vi "loggin'.vi"() -> ()   [LabVIEW 2018]
uses:
  <vilib>/Platform/TimedLoop/XDataNode/wakeup.ctl
  <vilib>/Platform/TimedLoop/XDataNode/XDNodeRunTimeDep.lvlib
  <vilib>/Platform/TimedLoop/XDataNode/nitl_modes.ctl
  <vilib>/Platform/TimedLoop/XDataNode/timing_clust.ctl
  <vilib>/platform/TimedLoop/XDataNode/XDataNode.xnode
  <userlib>/836-Library/System/QCP_V2/QCPSupportCode/QCPData.ctl
panel:
  out "QCP Finished Late? [i-1]":bool
  out "QCP Iteration Duration":i64=10
  in  "QCPPeriod":i64=100
  in  "DriveWriteQCPFile":bool
  in  "AutoWriteQCPFile":bool
  in  "HatchPanelWriteQCPFile":bool
  in  "ClimbWriteQCPFile":bool
  in  "CargoWriteQCPFile":bool
  in  "LiftTuningMode?":bool=TRUE
  in  "DriveTuningMode?":bool=TRUE
  in  "AutoTuningMode?":bool
  in  "IntakeTuningMode?":bool=TRUE
  in  "SensorTuningMode?":bool
  in  "Read Lift QCP":bool
  in  "Read Drive QCP":bool
  in  "Read Auto QCP":bool
  in  "Read Sensor QCP":bool
  in  "Read Intake QCP":bool
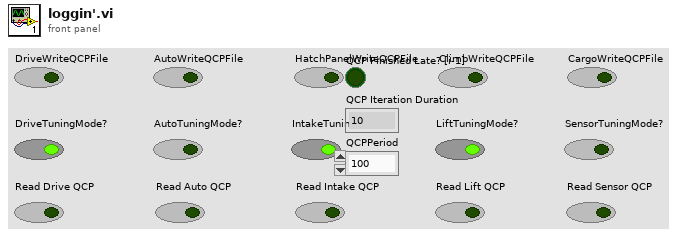
[diagram p1: front panel]
types:
  T1 = typedef "XDNodeRunTimeDep.lvlib/timing_clust.ctl" = cluster{"Expected End [f-1]":u64, "Actual End [f-1]":u64, "Finished Late? [f-1]":bool, "Expected End [i-1]":u64, "Actual End [i-1]":u64, "Finished Late? [i-1]":bool, "Expected Start [i]":u64, "Actual Start [i]":u64, "Expected Start [f]":u64, "Actual Start [f]":u64, "Source Name":string, "Structure Name":string, "Period":i64, "Deadline":i64, "Offset":i64, "Start":i64, "Priority":i32, "Timeout":i32, "Mode":T2, "Wakeup Reason":T3, "Error":errorcluster, "Source Type":string, "Secondary Source Type":string, "Global End Time":u64, "Global Start Time":u64, "Frame Duration":u64, "Iteration Duration":u64, "Assigned CPU":i32, "I/O Scan Engine Mode":u32}
  T2 = typedef "XDNodeRunTimeDep.lvlib/nitl_modes.ctl" = enum32{"No Change", "Process missed periods, maintain original phase", "Discard missed periods, maintain original phase", "Process missed periods, ignore original phase", "Discard missed periods, ignore original phase"}
  T3 = typedef "XDNodeRunTimeDep.lvlib/wakeup.ctl" = enum32{"Normal", "Aborted", "Asynchronous wakeup", "Timing source error", "Timed loop error", "Timeout"}
  T4 = typedef "Semaphore RefNum" = refnum<k1>
  T5 = cluster{"Data Value Refnum":refnum<data-value>, "semaphore":T4}
  T6 = typedef "QCP_RefNum.ctl" = cluster{"Data Value Refnum":refnum<data-value>, "semaphore":T4}
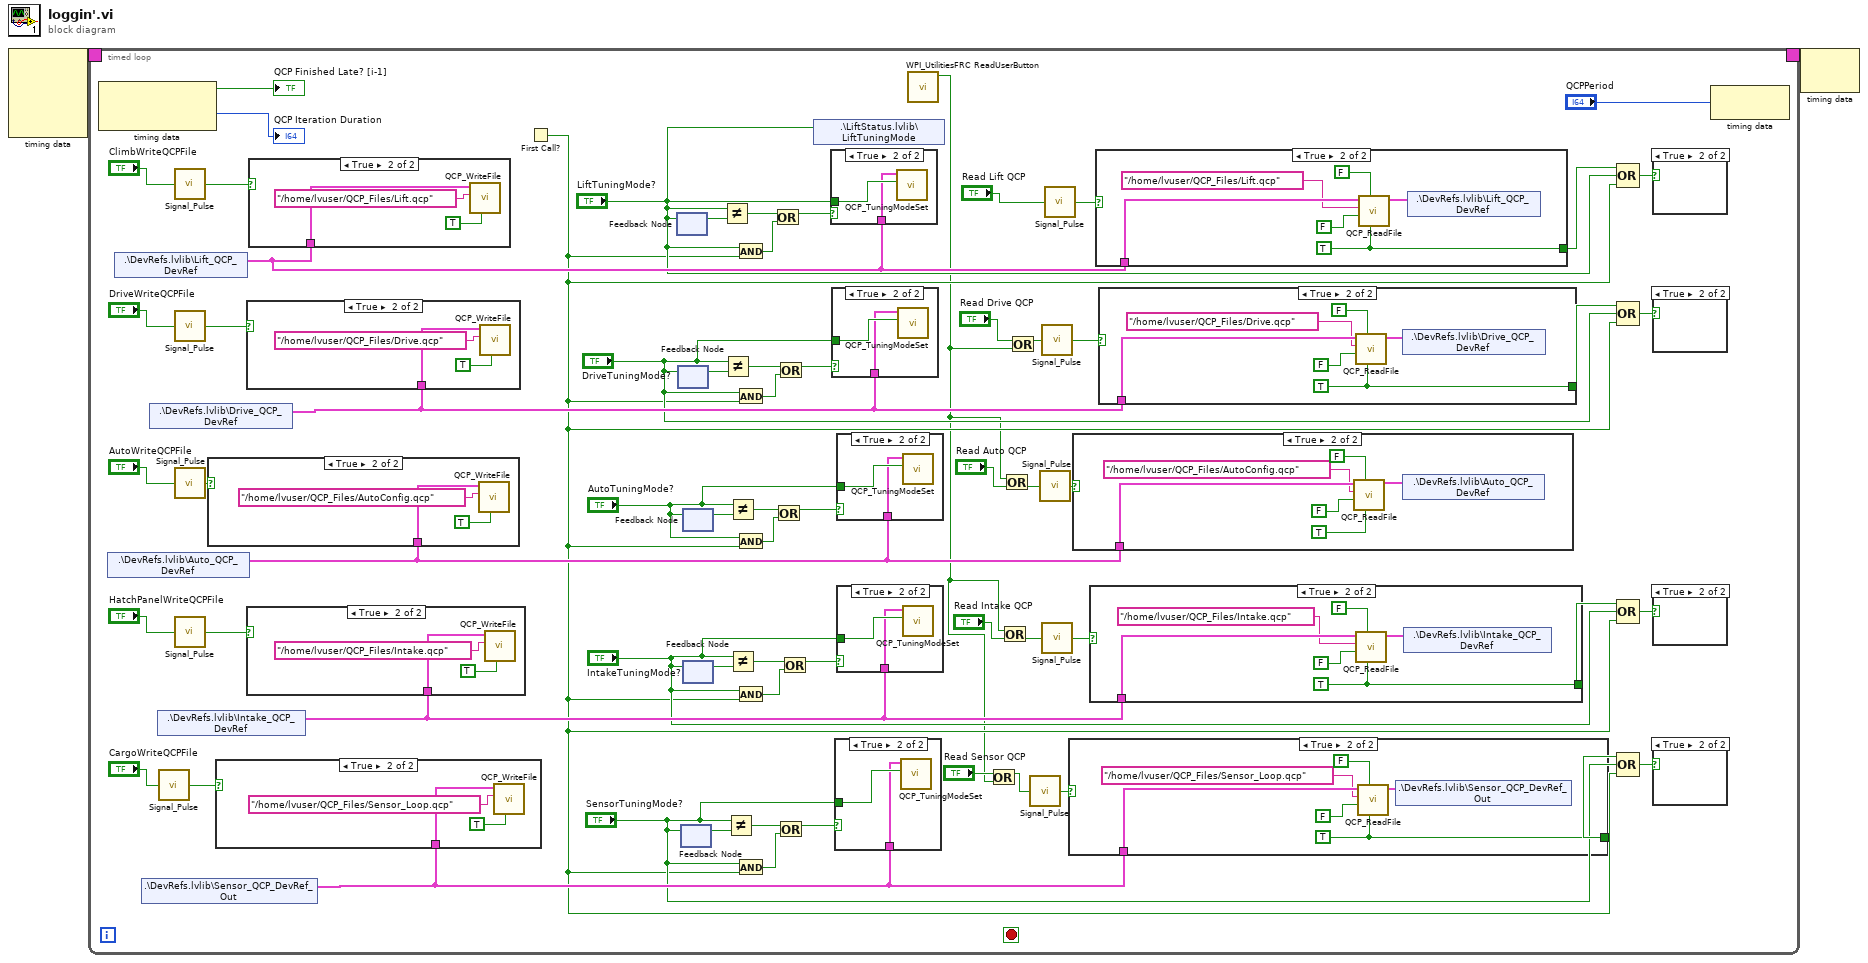
[diagram p0: block diagram]
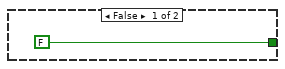
[diagram p6: hidden frame]
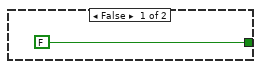
[diagram p7: hidden frame]
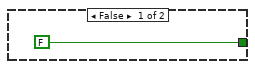
[diagram p9: hidden frame]
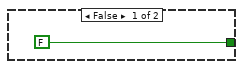
[diagram p10: hidden frame]
diagram:
  n1 = node-c288() -> (w2:T1)  [unwired: 4 in]
  n2 = timed-loop {
    timing: w2 -> [_]
    timing-out: [_] -> w1
    stop <- _ stop-if-true
    n3 = node-c288() -> (→"QCP Finished Late? [i-1]":bool, →"QCP Iteration Duration":i64)  [unwired: 1 in]
    n4 = shared-variable ".\\DevRefs.lvlib\\Auto_QCP_DevRef"() -> (w28:T5)  [unwired: 1 in, 1 out]
    n5 = shared-variable ".\\DevRefs.lvlib\\Lift_QCP_DevRef"() -> (w30:T5)  [unwired: 1 in, 1 out]
    n6 = shared-variable ".\\DevRefs.lvlib\\Sensor_QCP_DevRef_Out"() -> (w27:T5)  [unwired: 1 in, 1 out]
    n7 = shared-variable ".\\DevRefs.lvlib\\Drive_QCP_DevRef"() -> (w29:T5)  [unwired: 1 in, 1 out]
    n8 = shared-variable ".\\DevRefs.lvlib\\Intake_QCP_DevRef"() -> (w31:T5)  [unwired: 1 in, 1 out]
    n9 = call <userlib>:"Signal_Pulse.vi"("Input"="CargoWriteQCPFile") -> ("Output"=w58:bool)
    n10 = call <userlib>:"Signal_Pulse.vi"("Input"="ClimbWriteQCPFile") -> ("Output"=w60:bool)
    n11 = call <userlib>:"Signal_Pulse.vi"("Input"="DriveWriteQCPFile") -> ("Output"=w66:bool)
    n12 = call <userlib>:"Signal_Pulse.vi"("Input"="AutoWriteQCPFile") -> ("Output"=w64:bool)
    n13 = call <userlib>:"Signal_Pulse.vi"("Input"="HatchPanelWriteQCPFile") -> ("Output"=w62:bool)
    n14 = case shown="True" w64 {
      tunnel: w28 -> [_ w124]
      frame False {
      }
      frame True {
        n15 = call <userlib>:"QCP_WriteFile.vi"("Overrite?"=TRUE, "Path"="/home/lvuser/QCP_Files/AutoConfig.qcp", "QCP_DevRef_In"=w124) -> ()  [unwired: 7 in, 2 out]
      }
    }
    n16 = case shown="True" w58 {
      tunnel: w27 -> [_ w115]
      frame False {
      }
      frame True {
        n17 = call <userlib>:"QCP_WriteFile.vi"("Overrite?"=TRUE, "Path"="/home/lvuser/QCP_Files/Sensor_Loop.qcp", "QCP_DevRef_In"=w115) -> ()  [unwired: 7 in, 2 out]
      }
    }
    n18 = case shown="True" w66 {
      tunnel: w29 -> [_ w127]
      frame False {
      }
      frame True {
        n19 = call <userlib>:"QCP_WriteFile.vi"("Overrite?"=TRUE, "Path"="/home/lvuser/QCP_Files/Drive.qcp", "QCP_DevRef_In"=w127) -> ()  [unwired: 7 in, 2 out]
      }
    }
    n20 = case shown="True" w62 {
      tunnel: w31 -> [_ w121]
      frame False {
      }
      frame True {
        n21 = call <userlib>:"QCP_WriteFile.vi"("Overrite?"=TRUE, "Path"="/home/lvuser/QCP_Files/Intake.qcp", "QCP_DevRef_In"=w121) -> ()  [unwired: 7 in, 2 out]
      }
    }
    n22 = case shown="True" w60 {
      tunnel: w30 -> [_ w118]
      frame False {
      }
      frame True {
        n23 = call <userlib>:"QCP_WriteFile.vi"("Overrite?"=TRUE, "Path"="/home/lvuser/QCP_Files/Lift.qcp", "QCP_DevRef_In"=w118) -> ()  [unwired: 7 in, 2 out]
      }
    }
    n24 = First Call?() -> (First Call?: T/F=w10:bool)
    n25 = feedback #1() -> (w56:bool)  [unwired: 1 in]
    n26 = feedback-in #1("LiftTuningMode?") -> ()
    n27 = feedback #2() -> (w55:bool)  [unwired: 1 in]
    n28 = feedback-in #2("DriveTuningMode?") -> ()
    n29 = feedback #3() -> (w49:bool)  [unwired: 1 in]
    n30 = feedback-in #3("SensorTuningMode?") -> ()
    n31 = feedback #4() -> (w53:bool)  [unwired: 1 in]
    n32 = feedback-in #4("AutoTuningMode?") -> ()
    n33 = feedback #5() -> (w51:bool)  [unwired: 1 in]
    n34 = feedback-in #5("IntakeTuningMode?") -> ()
    n35 = Not Equal?(x="LiftTuningMode?", y=w56) -> (x != y?=w21:bool)
    n36 = Not Equal?(x="DriveTuningMode?", y=w55) -> (x != y?=w54:bool)
    n37 = Not Equal?(x="SensorTuningMode?", y=w49) -> (x != y?=w48:bool)
    n38 = Not Equal?(x="AutoTuningMode?", y=w53) -> (x != y?=w52:bool)
    n39 = Not Equal?(x="IntakeTuningMode?", y=w51) -> (x != y?=w50:bool)
    n40 = And(x="LiftTuningMode?", y=w10) -> (x .and. y?=w20:bool)
    n41 = And(x="DriveTuningMode?", y=w10) -> (x .and. y?=w18:bool)
    n42 = And(x="AutoTuningMode?", y=w10) -> (x .and. y?=w11:bool)
    n43 = And(x="IntakeTuningMode?", y=w10) -> (x .and. y?=w15:bool)
    n44 = And(x="SensorTuningMode?", y=w10) -> (x .and. y?=w13:bool)
    n45 = Or(x=w21, y=w20) -> (x .or. y?=w22:bool)
    n46 = Or(x=w52, y=w11) -> (x .or. y?=w24:bool)
    n47 = Or(x=w54, y=w18) -> (x .or. y?=w23:bool)
    n48 = Or(x=w48, y=w13) -> (x .or. y?=w26:bool)
    n49 = Or(x=w50, y=w15) -> (x .or. y?=w25:bool)
    n50 = shared-variable ".\\LiftStatus.lvlib\\LiftTuningMode"("LiftTuningMode?") -> ()  [unwired: 1 in, 1 out]
    n51 = case shown="True" w22 {
      tunnel: "LiftTuningMode?" -> [_ w113]
      tunnel: w30 -> [_ w112]
      frame False {
      }
      frame True {
        n52 = call <userlib>:"QCP_TuningModeSet.vi"("On?"=w113, "QCP_DevRef_In"=w112) -> ()  [unwired: 8 in, 2 out]
      }
    }
    n53 = case shown="True" w23 {
      tunnel: "DriveTuningMode?" -> [_ w111]
      tunnel: w29 -> [_ w110]
      frame False {
      }
      frame True {
        n54 = call <userlib>:"QCP_TuningModeSet.vi"("On?"=w111, "QCP_DevRef_In"=w110) -> ()  [unwired: 8 in, 2 out]
      }
    }
    n55 = case shown="True" w26 {
      tunnel: "SensorTuningMode?" -> [_ w105]
      tunnel: w27 -> [_ w104]
      frame False {
      }
      frame True {
        n56 = call <userlib>:"QCP_TuningModeSet.vi"("On?"=w105, "QCP_DevRef_In"=w104) -> ()  [unwired: 8 in, 2 out]
      }
    }
    n57 = case shown="True" w24 {
      tunnel: "AutoTuningMode?" -> [_ w109]
      tunnel: w28 -> [_ w108]
      frame False {
      }
      frame True {
        n58 = call <userlib>:"QCP_TuningModeSet.vi"("On?"=w109, "QCP_DevRef_In"=w108) -> ()  [unwired: 8 in, 2 out]
      }
    }
    n59 = case shown="True" w25 {
      tunnel: "IntakeTuningMode?" -> [_ w107]
      tunnel: w31 -> [_ w106]
      frame False {
      }
      frame True {
        n60 = call <userlib>:"QCP_TuningModeSet.vi"("On?"=w107, "QCP_DevRef_In"=w106) -> ()  [unwired: 8 in, 2 out]
      }
    }
    n61 = call <vilib>:"WPI_UtilitiesFRC ReadUserButton.vi"() -> ("User Button"=w4:bool)  [unwired: 10 in, 1 out]
    n62 = Or(x="Read Sensor QCP", y=w4) -> (x .or. y?=w5:bool)
    n63 = Or(x=w4, y="Read Intake QCP") -> (x .or. y?=w6:bool)
    n64 = Or(x=w4, y="Read Auto QCP") -> (x .or. y?=w7:bool)
    n65 = Or(x="Read Drive QCP", y=w4) -> (x .or. y?=w9:bool)
    n66 = call <userlib>:"Signal_Pulse.vi"("Input"=w5) -> ("Output"=w43:bool)
    n67 = call <userlib>:"Signal_Pulse.vi"("Input"=w7) -> ("Output"=w45:bool)
    n68 = call <userlib>:"Signal_Pulse.vi"("Input"=w9) -> ("Output"=w46:bool)
    n69 = call <userlib>:"Signal_Pulse.vi"("Input"=w6) -> ("Output"=w44:bool)
    n70 = call <userlib>:"Signal_Pulse.vi"("Input"="Read Lift QCP") -> ("Output"=w47:bool)
    n71 = case shown="True" w43 {
      tunnel: w27 -> [_ w76]
      tunnel: [FALSE ("Overrite Existing Data?") w72] -> w36
      frame False {
      }
      frame True {
        w72 = TRUE ("Overrite Existing Data?")
        n72 = call <userlib>:"QCP_ReadFile.vi"("Overrite Existing Data?"=w72, "Same Name Fail?"=FALSE, "Path Relative?"=FALSE, "Path"="/home/lvuser/QCP_Files/Sensor_Loop.qcp", "QCP_DevRef_In"=w76) -> ("QCP_DevRef_Out"=w71:T6)  [unwired: 5 in, 1 out]
        n73 = shared-variable ".\\DevRefs.lvlib\\Sensor_QCP_DevRef_Out"(w71) -> ()  [unwired: 1 in, 1 out]
      }
    }
    n74 = case shown="True" w45 {
      tunnel: w28 -> [_ w89]
      frame False {
      }
      frame True {
        n75 = call <userlib>:"QCP_ReadFile.vi"("Overrite Existing Data?"=TRUE, "Same Name Fail?"=FALSE, "Path Relative?"=FALSE, "Path"="/home/lvuser/QCP_Files/AutoConfig.qcp", "QCP_DevRef_In"=w89) -> ("QCP_DevRef_Out"=w84:T6)  [unwired: 5 in, 1 out]
        n76 = shared-variable ".\\DevRefs.lvlib\\Auto_QCP_DevRef"(w84) -> ()  [unwired: 1 in, 1 out]
      }
    }
    n77 = case shown="True" w44 {
      tunnel: w31 -> [_ w83]
      tunnel: [FALSE ("Overrite Existing Data?") w79] -> w38
      frame False {
      }
      frame True {
        w79 = TRUE ("Overrite Existing Data?")
        n78 = call <userlib>:"QCP_ReadFile.vi"("Overrite Existing Data?"=w79, "Same Name Fail?"=FALSE, "Path Relative?"=FALSE, "Path"="/home/lvuser/QCP_Files/Intake.qcp", "QCP_DevRef_In"=w83) -> ("QCP_DevRef_Out"=w78:T6)  [unwired: 5 in, 1 out]
        n79 = shared-variable ".\\DevRefs.lvlib\\Intake_QCP_DevRef"(w78) -> ()  [unwired: 1 in, 1 out]
      }
    }
    n80 = case shown="True" w47 {
      tunnel: w30 -> [_ w103]
      tunnel: [FALSE ("Overrite Existing Data?") w99] -> w32
      frame False {
      }
      frame True {
        w99 = TRUE ("Overrite Existing Data?")
        n81 = call <userlib>:"QCP_ReadFile.vi"("Overrite Existing Data?"=w99, "Same Name Fail?"=FALSE, "Path Relative?"=FALSE, "Path"="/home/lvuser/QCP_Files/Lift.qcp", "QCP_DevRef_In"=w103) -> ("QCP_DevRef_Out"=w98:T6)  [unwired: 5 in, 1 out]
        n82 = shared-variable ".\\DevRefs.lvlib\\Lift_QCP_DevRef"(w98) -> ()  [unwired: 1 in, 1 out]
      }
    }
    n83 = case shown="True" w46 {
      tunnel: w29 -> [_ w96]
      tunnel: [FALSE ("Overrite Existing Data?") w92] -> w34
      frame False {
      }
      frame True {
        w92 = TRUE ("Overrite Existing Data?")
        n84 = call <userlib>:"QCP_ReadFile.vi"("Overrite Existing Data?"=w92, "Same Name Fail?"=FALSE, "Path Relative?"=FALSE, "Path"="/home/lvuser/QCP_Files/Drive.qcp", "QCP_DevRef_In"=w96) -> ("QCP_DevRef_Out"=w91:T6)  [unwired: 5 in, 1 out]
        n85 = shared-variable ".\\DevRefs.lvlib\\Drive_QCP_DevRef"(w91) -> ()  [unwired: 1 in, 1 out]
      }
    }
    n86 = Compound Arithmetic op=OR(w32, "LiftTuningMode?", w10) -> (w33:bool)
    n87 = Compound Arithmetic op=OR(w34, "DriveTuningMode?", w10) -> (w35:bool)
    n88 = Compound Arithmetic op=OR(w38, "IntakeTuningMode?", w10) -> (w39:bool)
    n89 = Compound Arithmetic op=OR(w36, "SensorTuningMode?", w10) -> (w37:bool)
    n90 = case shown="True" w33 {
      frame False {
      }
      frame True {
      }
    }
    n91 = case shown="True" w35 {
      frame False {
      }
      frame True {
      }
    }
    n92 = case shown="True" w39 {
      frame False {
      }
      frame True {
      }
    }
    n93 = case shown="True" w37 {
      frame False {
      }
      frame True {
      }
    }
    n94 = node-c288("QCPPeriod") -> ()  [unwired: 1 out]
  }
  n95 = node-c288(w1) -> ()  [unwired: 1 out]
